vi "Stop Nested Actors.vi"(8 "error in":errorcluster, 11 "Controller in":refnum<class "Controller.lvclass">) -> (0 "error out":errorcluster, 3 "Controller out":refnum<class "Controller.lvclass">)   [LabVIEW 2014, in "Controller.lvlib" / "Controller.lvclass"]
uses:
  Controller.lvclass
  Controls/eMap.ctl
  <vilib>/ActorFramework/Message Enqueuer/Message Enqueuer.lvclass
  Controller.lvclass/Controller.ctl
  <vilib>/ActorFramework/Message Enqueuer/Message Enqueuer.lvclass/Message Enqueuer.ctl
  <vilib>/ActorFramework/Message Enqueuer/Enqueue.vi
  <vilib>/ActorFramework/Message Priority Queue/Priority Enqueue.vi
  <vilib>/ActorFramework/Stop Msg/Stop Msg.lvclass
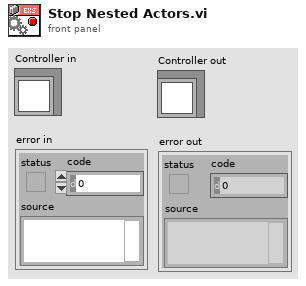
[diagram p1: front panel]
types:
  T1 = typedef "Controller.lvlib/Controller.lvclass/eMap.ctl" = cluster{"Enqueuer":refnum<class "Message Enqueuer.lvclass">, "Active":bool}
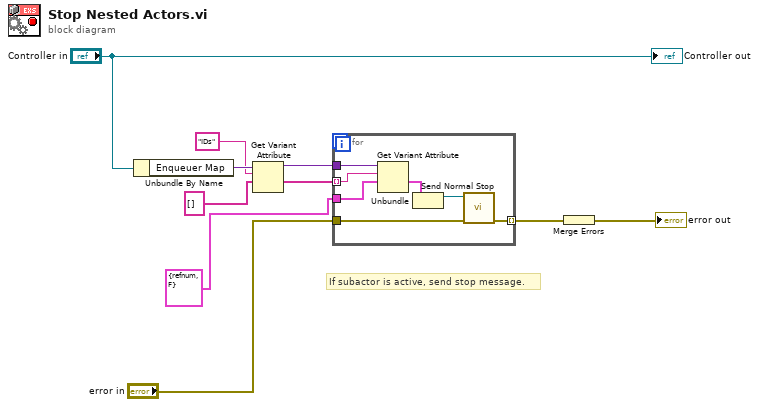
[diagram p0: block diagram]
diagram:
  # "If subactor is active, send stop message."
  n1 = Unbundle By Name("Controller in") -> ("Enqueuer Map"=w8:variant)
  n2 = Get Variant Attribute(Variant=w8, name="IDs", default value (empty Variant)=string[] []) -> (duplicate Variant=w4:variant, value=w5:string[])  [unwired: 1 in, 2 out]
  n3 = for {
    tunnel: "error in" -> [w17]
    tunnel: [w16] -> w2 mode=indexing
    tunnel: w5 -> [w14] mode=indexing
    tunnel: w4 -> [w15]
    tunnel: T1 {"Enqueuer"=refnum, "Active"=FALSE} ("eMap") -> [w13]
    n4 = Get Variant Attribute(Variant=w15, name=w14, default value (empty Variant)=w13) -> (value=w12:T1)  [unwired: 1 in, 3 out]
    n5 = Unbundle(w12) -> ("Enqueuer"=w11:refnum<class "Message Enqueuer.lvclass">)  [unwired: 1 out]
    n6 = call <vilib>:"Send Normal Stop.vi"("error in (no error)"=w17, "Message Enqueuer"=w11) -> ("error out"=w16:errorcluster)  [unwired: 9 in]
  }
  n7 = Merge Errors(w2) -> (→"error out":errorcluster)
  "Controller out" <- "Controller in"
